vi "ziModGetNodeValueDouble.vi"(0 "ModHandle In":T1 {"ModHandle" format="0x%08x"; "Conn" format="0x%08x"}, 7 "Path":string, 11 "error in":errorcluster) -> (4 "ModHandle Out":T1 {"ModHandle" format="0x%08x"; "Conn" format="0x%08x"}, 8 "Value":dbl, 15 "error out":errorcluster)   [LabVIEW 2018, in "Zurich Instruments LabOne.lvlib"]
doc: "FOR MODULES This vi retrieves the numerical value of the specified node as an double-type value. The vi returns the value first found that matches Path if more than one value is available (a wildcard is used in the Path)."
uses:
  Zurich Instruments LabOne.lvlib
  ziTypeModHandle.ctl
  ziLV32.dll
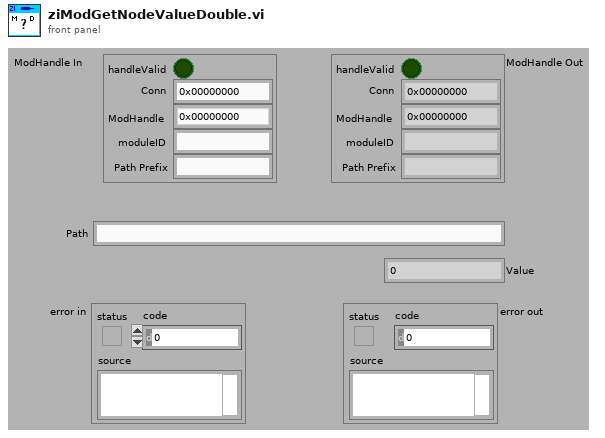
[diagram p1: front panel]
types:
  T1 = typedef "Zurich Instruments LabOne.lvlib/ziTypeModHandle.ctl" = cluster{"handleValid":bool, "Conn":u64, "ModHandle":u64, "moduleID":string, "Path Prefix":string}
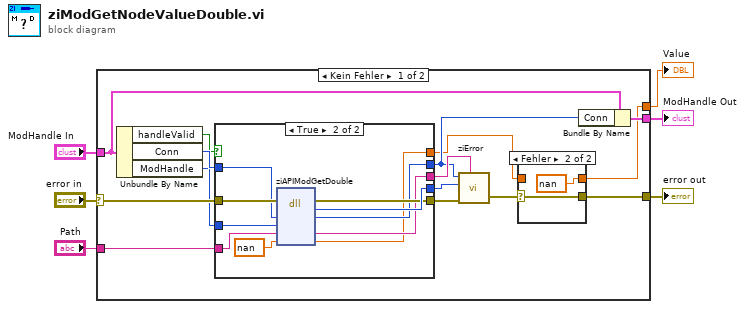
[diagram p0: block diagram]
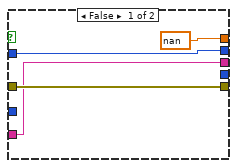
[diagram p3: hidden frame]
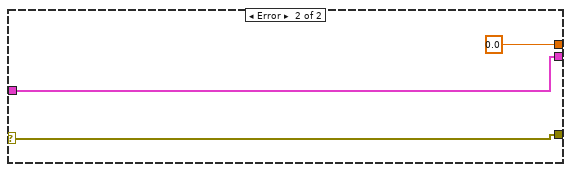
[diagram p4: hidden frame]
diagram:
  n1 = case shown="Kein Fehler" "error in" {
    selector: "error in" -> [w18 w42]
    tunnel: [w7 w42] -> w6
    tunnel: [w19 w41] -> w2
    tunnel: "ModHandle In" -> [w13 w41]
    tunnel: "Path" -> [w14 _]
    tunnel: [w9 0.0 ("Value")] -> w1
    frame No Error {
      n2 = Unbundle By Name(w13) -> ("handleValid"=w11:bool, "Conn"=w16:u64, "ModHandle"=w12:u64)
      n3 = case shown="True" w11 {
        tunnel: [_ w39] -> w21
        tunnel: [w29 w38] -> w20
        tunnel: w18 -> [w29 w37]
        tunnel: [w27 w36] -> w17
        tunnel: w16 -> [w28 w35]
        tunnel: [w28 w34] -> w15
        tunnel: w14 -> [w27 w33]
        tunnel: w12 -> [_ w32]
        tunnel: [nan ("Value") w30] -> w10
        frame False {
        }
        frame True {
          n4 = dll-call lib="ziLV*.*" fn="ziAPIModGetDouble"(error in=w37, "Conn"=w35, "ModHandle"=w32, "Path"=w33, "Value"=nan) -> (error out=w38:errorcluster, "return type"=w39:u32, "Conn"=w34:u64, "Path"=w36:string, "Value"=w30:dbl)  [unwired: 3 in, 1 out]
        }
      }
      n5 = call "ziError.vi"("Conn"=w15, "ziErrorCode"=w21, "Error In"=w20, "Annotation"=w17) -> ("Error Out"=w8:errorcluster)  [unwired: 2 in]
      n6 = case shown="Fehler" w8 {
        selector: w8 -> [w22 w24]
        tunnel: w10 -> [w23 _]
        tunnel: [w23 nan ("Value")] -> w9
        tunnel: [w22 w24] -> w7
        frame No Error {
        }
        frame Error {
        }
      }
      n7 = Bundle By Name(cluster=w13, "Conn"=w15) -> (w19:T1)
    }
    frame Error {
    }
  }
  "error out" <- w6
  "Value" <- w1
  "ModHandle Out" <- w2
